vi "队列组.vi"(8 "错误输入（无错误）":errorcluster, 11 "队列名称":string[](array[string])) -> (0 "错误输出":errorcluster, 3 "队列组":refnum<queue>[](array[refnum]))   [LabVIEW 2021, in "QueueLib.lvlib"]
uses:
  QueueLib.lvlib
  <vilib>/Utility/error.llb/Error Cluster From Error Code.vi
  <vilib>/ErrorRing/Error Ring.xnode
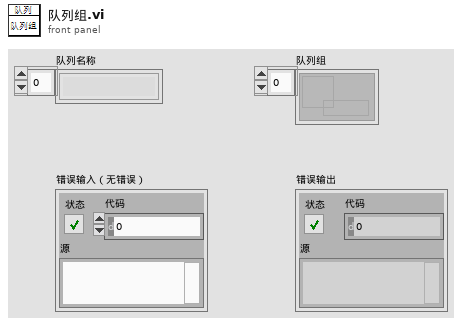
[diagram p1: front panel]
types:
  T1 = typedef "QueueLib.lvlib/数据类型.ctl" = cluster{"消息":string, "数据":variant}
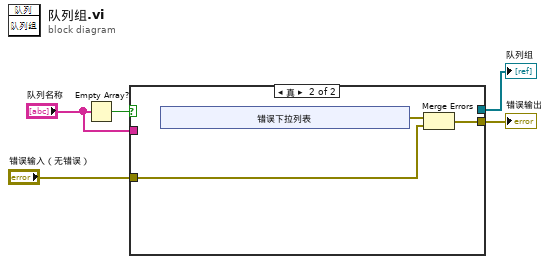
[diagram p0: block diagram]
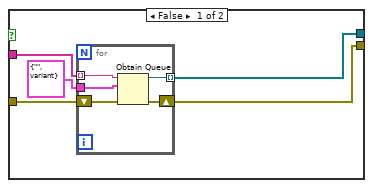
[diagram p2: hidden frame]
diagram:
  n1 = Empty Array?(array="队列名称") -> (empty?=w2:bool)
  n2 = case shown="真" w2 {
    tunnel: [w10 _] -> w1
    tunnel: [w9 w16] -> w5
    tunnel: "错误输入（无错误）" -> [w8 w18]
    tunnel: "队列名称" -> [w7 _]
    frame False {
      n3 = for {
        tunnel: T1 {"消息"="", "数据"=variant} ("数据类型") -> [w15]
        tunnel: w7 -> [w13] mode=indexing
        shift-right: [w11] -> w9
        shift-left: w8 -> [w14]
        tunnel: [w12] -> w10 mode=indexing
        n4 = Obtain Queue(name (unnamed)=w13, element data type=w15, error in (no error)=w14) -> (queue out=w12:refnum<queue>, error out=w11:errorcluster)  [unwired: 2 in, 1 out]
      }
    }
    frame True {
      n5 = xnode "错误下拉列表"() -> ("错误输出"=w17:errorcluster)
      n6 = Merge Errors(w17, w18) -> (w16:errorcluster)
    }
  }
  "错误输出" <- w5
  "队列组" <- w1
